vi "SetupDefault.vi"(8 "error in (no error)":errorcluster, 11 "NetA_AgNA in":refnum<class "NetA_AgNA.lvclass">) -> (0 "error out":errorcluster, 3 "NetA_AgNA out":refnum<class "NetA_AgNA.lvclass">)   [LabVIEW 2014, in "NetA_AgNA.lvclass"]
uses:
  NetA_AgNA.lvclass
  NetA_AgNA.lvclass/NetA_AgNA.ctl
panel:
  in  "Alias":string
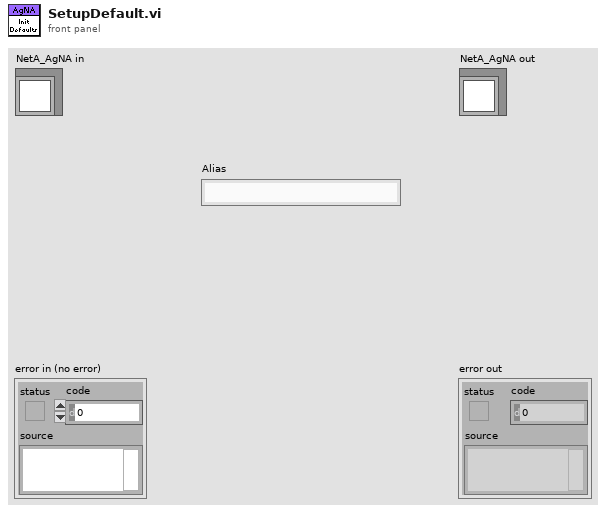
[diagram p1: front panel]
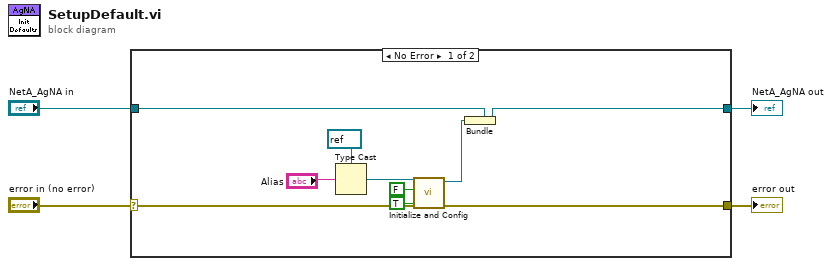
[diagram p0: block diagram]
diagram:
  n1 = case shown="No Error" "error in (no error)" {
    selector: "error in (no error)" -> [w13 w16]
    tunnel: [w12 w16] -> w3
    tunnel: [w10 w15] -> w1
    tunnel: "NetA_AgNA in" -> [w14 w15]
    frame No Error {
      n2 = Type Cast(type=refnum<k15> refnum ("instrument handle out"), x="Alias") -> (*(type *) &x=w5:refnum<k15>)
      n3 = call "Initialize and Config.vi"("error in (no error)"=w13, "reset device (Off)"=TRUE, "id query (Off)"=FALSE, "NETAN"=w5) -> ("error out"=w12:errorcluster, "instrument handle out"=w9:refnum<k15>)  [unwired: 6 in]
      n4 = Bundle(cluster=w14, w9) -> (w10:refnum<class "NetA_AgNA.lvclass">)
    }
    frame Error {
    }
  }
  "error out" <- w3
  "NetA_AgNA out" <- w1
